vi "lorentzian transformations.vi"(6 "factor":dbl=1.0, 7 "4 corner circle transformation":T3=enum."fix phase", 8 "lorentzian in":T2 {"z∞ (V)" format="%#_4p"; "Q" format="%#_4p"; "φ (rad)" format="%#_3p"; "Γ (Hz)" format="%#_5p"; "ω (Hz)" format="%#_9p"; "A (VHz)" format="%#_3p"}, 9 "phase in (rad)":dbl, 10 "freq in":dbl, 11 "voltage in":cdb) -> (0 "lorentzian out":T2={"A (VHz)"=-1.0311345636926572, "ω (Hz)"=-1.0311345636926572, "Γ (Hz)"=-1.0311345636926572, "φ (rad)"=-1.0311345636926572, "Q"=-1.0311345636926572, "Norm  Ampl"=-1.0311345636926572, "z∞ (V)"=-1.0311345636926572+0.0i, "4corners"={"z (-pi/2)"=-1.0311345636926572+0.5736824521422934i, "z(inf)"=-0.5200164984937075+1.0975277942502903i, "z (pi/2)"=-1.0311345636926572+0.5736824521422934i, "z center"=-0.5136528600391839+0.580046090596817i, "z(0)"=-0.5200164984937075+1.0975277942502903i, "radius"=-1.0311345636926572}} {"z∞ (V)" format="%#_4p"; "Q" format="%#_4p"; "φ (rad)" format="%#_3p"; "Γ (Hz)" format="%#_5p"; "ω (Hz)" format="%#_9p"; "A (VHz)" format="%#_3p"}, 1 "4corners our":T1={"z (-pi/2)"=-1.0311345636926572+0.5736824521422934i, "z(inf)"=-0.5200164984937075+1.0975277942502903i, "z (pi/2)"=-1.0311345636926572+0.5736824521422934i, "z center"=-0.5136528600391839+0.580046090596817i, "z(0)"=-0.5200164984937075+1.0975277942502903i, "radius"=-1.0311345636926572}, 2 "gamma OUT":dbl, 3 "voltage out":cdb)   [LabVIEW 2020]
uses:
  four-corner circle transformation.ctl
  lorentzian.ctl
  circle corners.ctl
  Q - not nan -- real.vi
panel:
  out "freq OUT":dbl
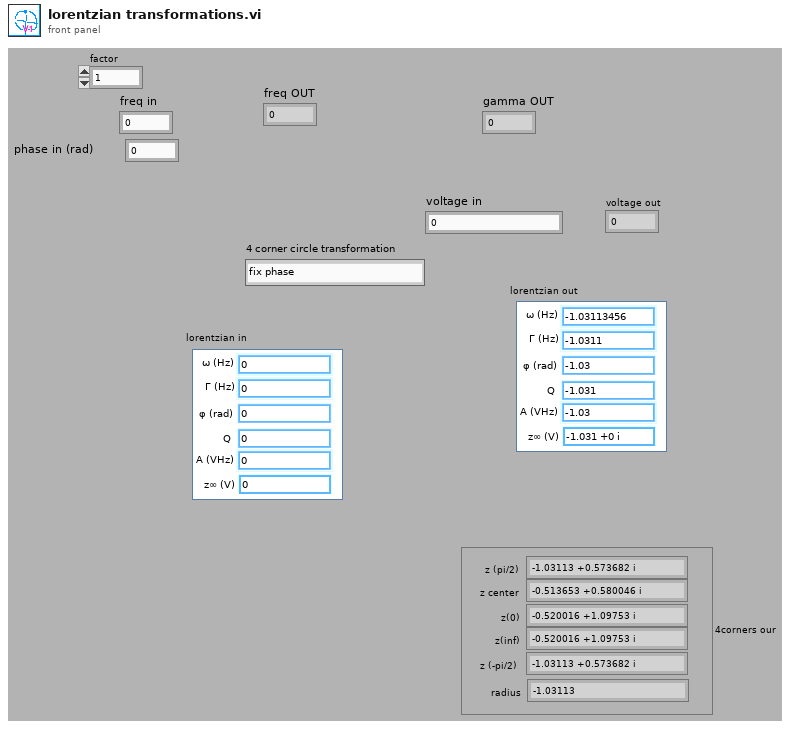
[diagram p1: front panel]
types:
  T1 = typedef "circle corners.ctl" = cluster{"z (-pi/2)":cdb, "z(inf)":cdb, "z (pi/2)":cdb, "z center":cdb, "z(0)":cdb, "radius":dbl}
  T2 = typedef "lorentzian.ctl" = cluster{"A (VHz)":dbl, "ω (Hz)":dbl, "Γ (Hz)":dbl, "φ (rad)":dbl, "Q":dbl, "Norm  Ampl":dbl, "z∞ (V)":cdb, "4corners":T1}
  T3 = typedef "four-corner circle transformation.ctl" = enum16{"z(c) z(inf)", "z(c) z(zero)", "fix phase", "calculate lorentzian", "z(0) z(+-pi/2)", "shift to zcenter", "to  canonical", "get canonical phase", "get4corners", "update lorentzian -- from z0", "fake gamma normal", "fake gamma heat", "calculate complex slope", "get f0 given f and phi"}
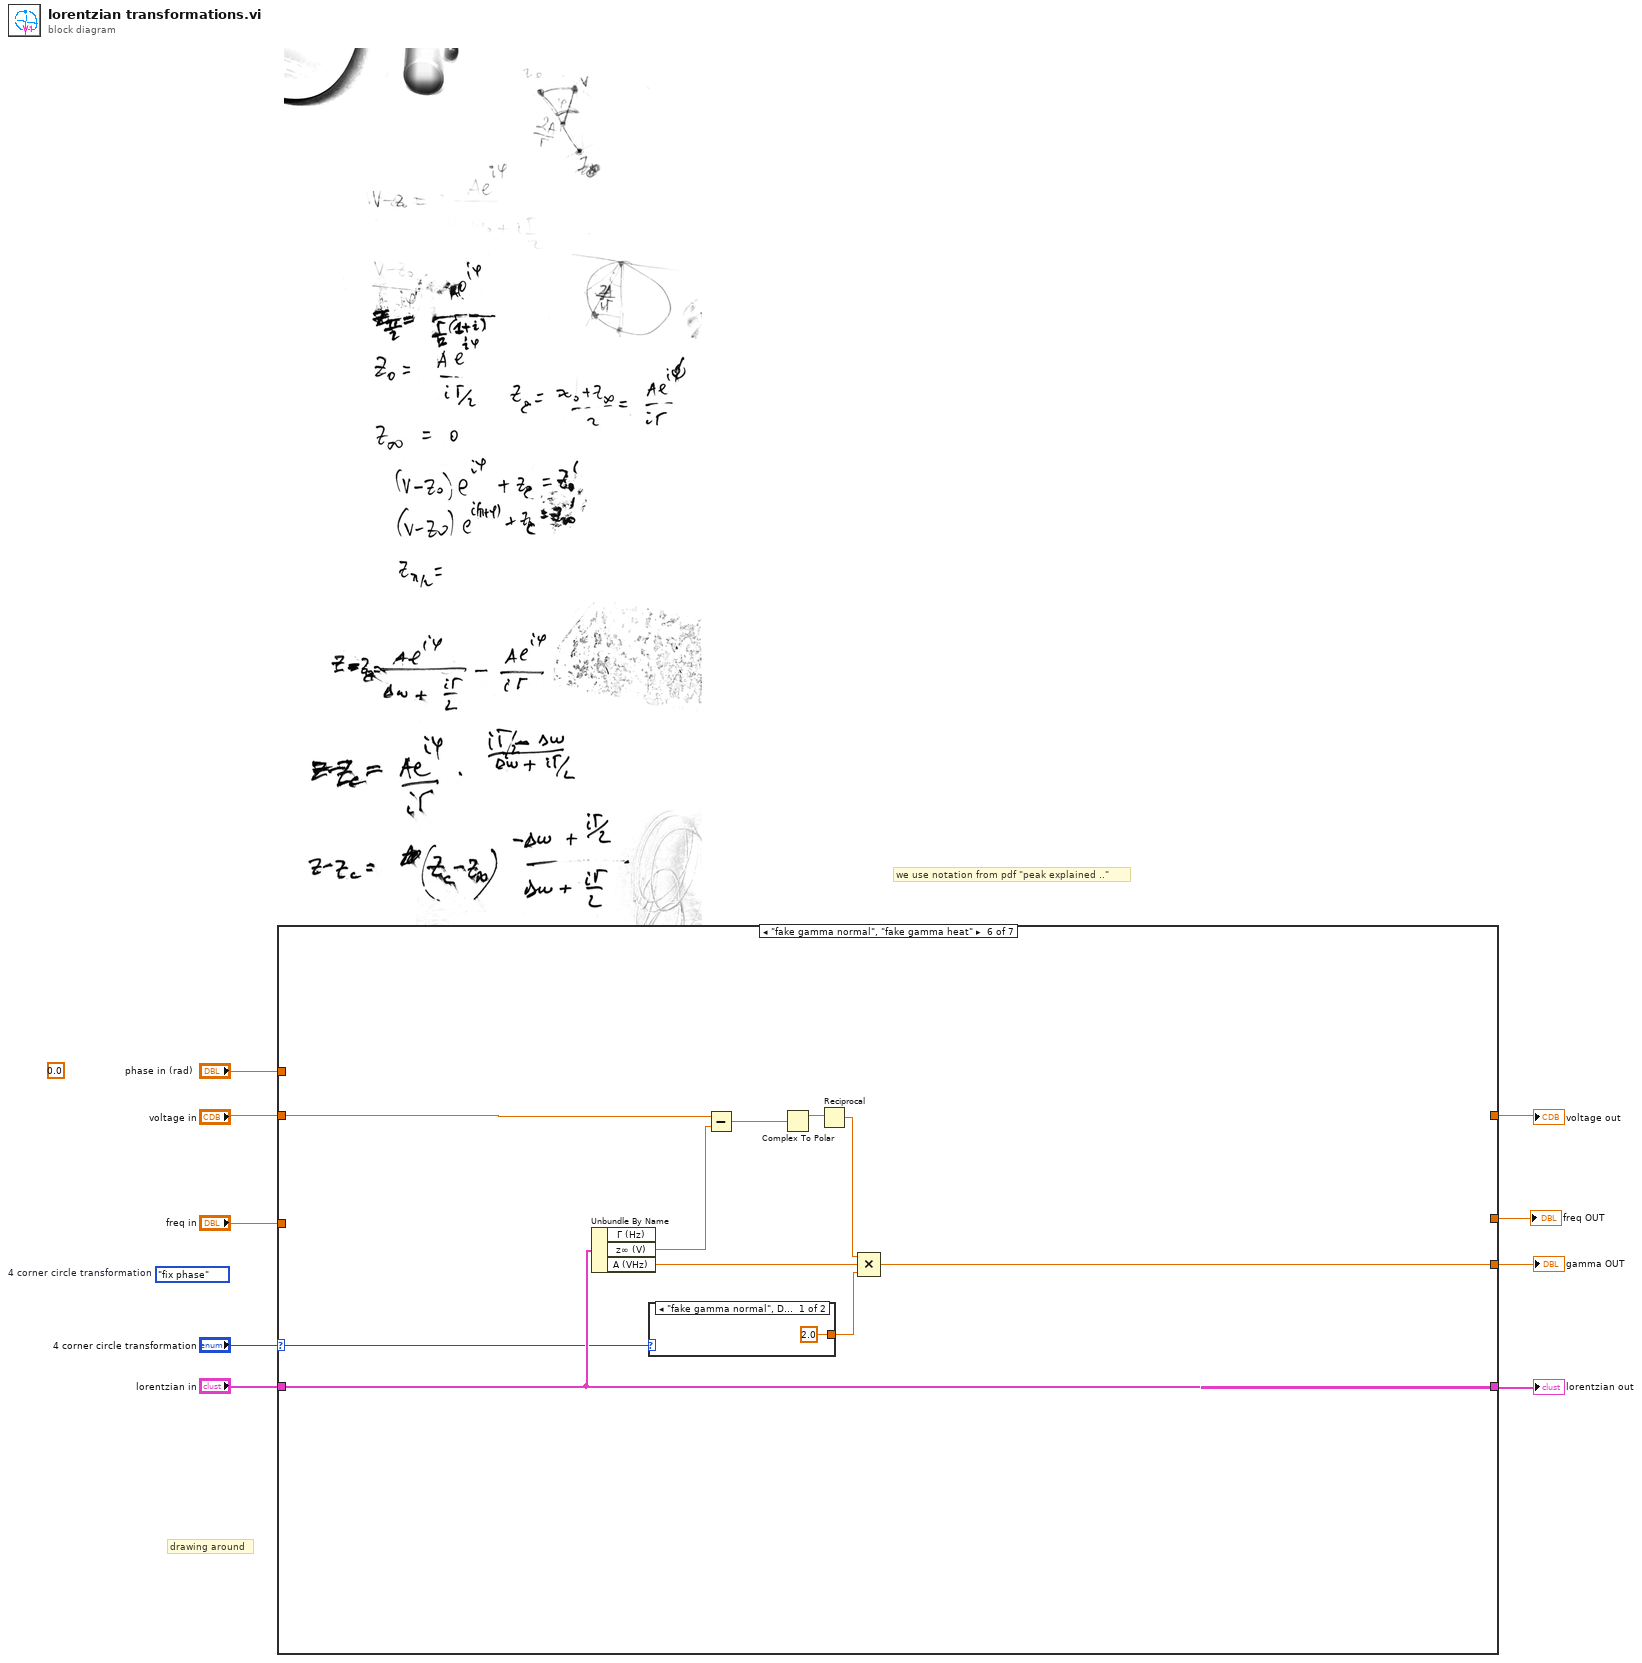
[diagram p0: block diagram]
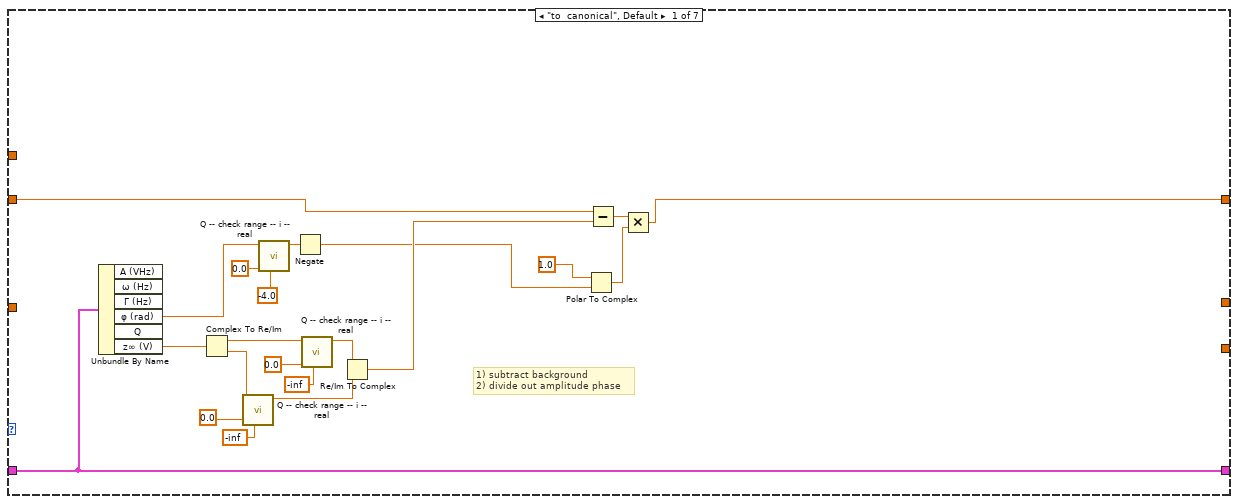
[diagram p2: hidden frame]
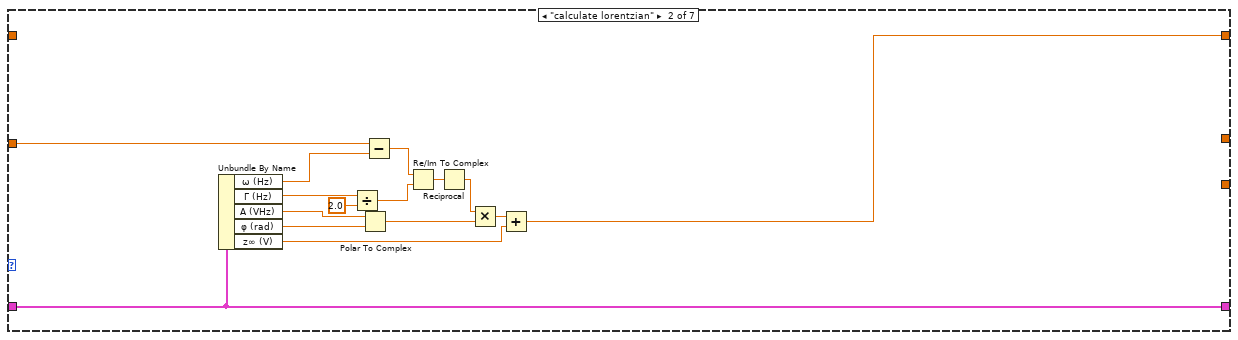
[diagram p3: hidden frame]
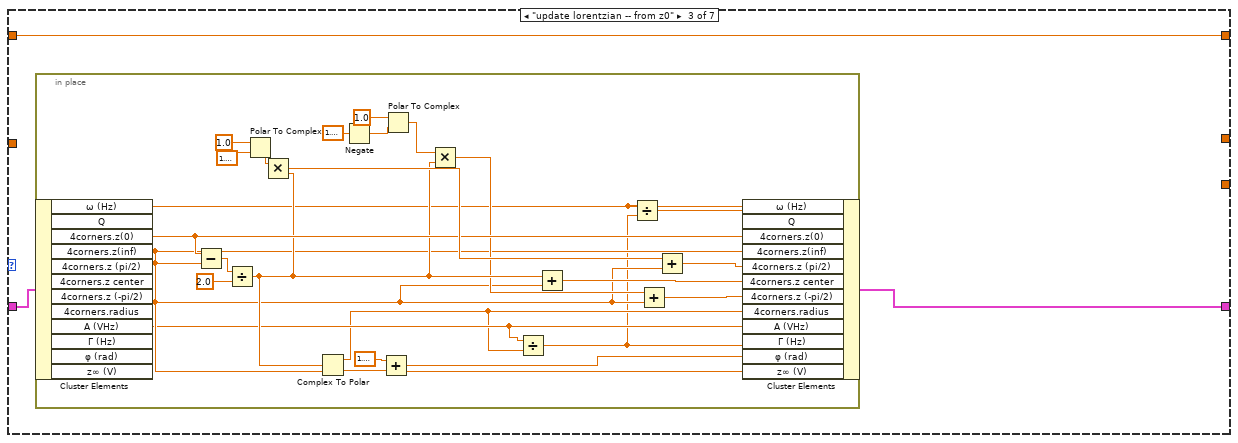
[diagram p4: hidden frame]
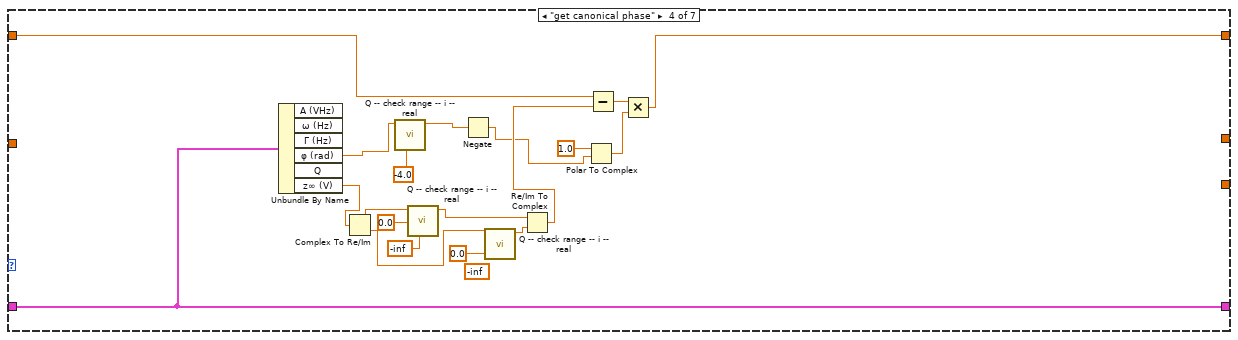
[diagram p5: hidden frame]
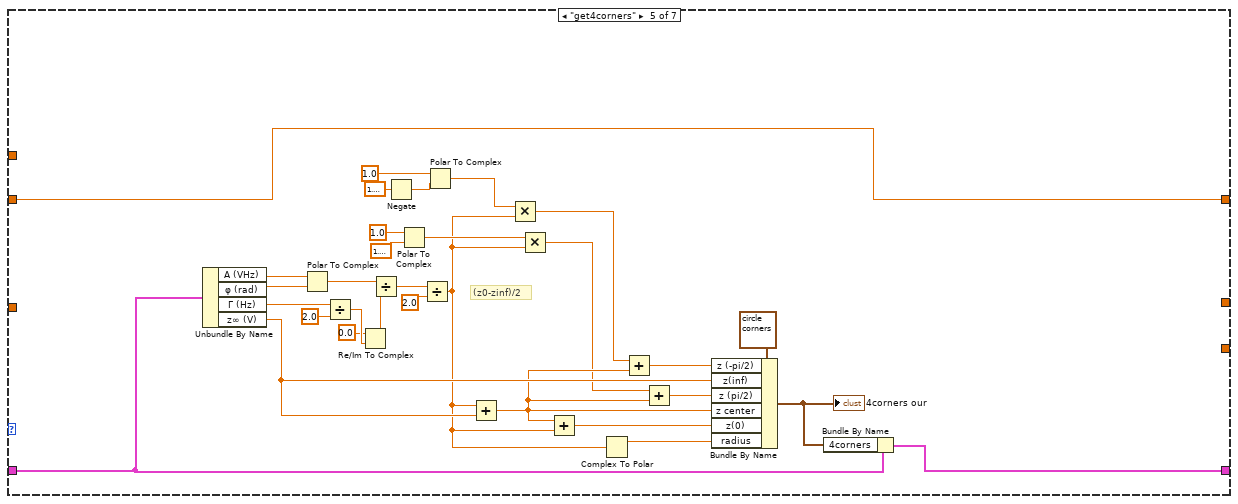
[diagram p6: hidden frame]
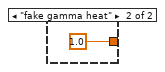
[diagram p7: hidden frame]
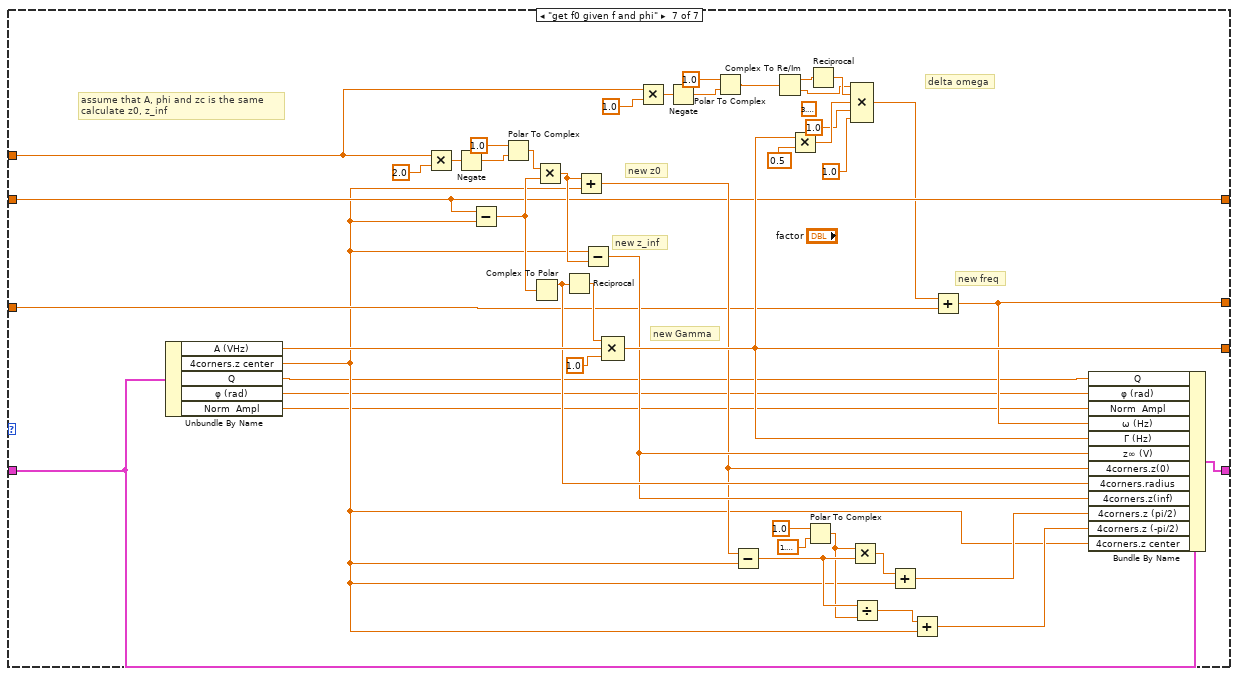
[diagram p8: hidden frame]
diagram:
  (unwired) 0.0 ("zi phase temporary")
  (unwired) four-corner_circle_transformation."fix phase"  # 4 corner circle transformation
  # "we use notation from pdf \"peak explained ..\""
  # "drawing around"
  n1 = case shown="\"fake gamma normal\", \"fake gamma heat\"" "4 corner circle transformation" {
    selector: "4 corner circle transformation" -> [_ _ _ _ _ w124 _]
    tunnel: "voltage in" -> [w13 _ w46 w75 w102 w127 w153]
    tunnel: [w14 w45 w47 w76 w95 w126 w171] -> w7
    tunnel: "lorentzian in" -> [w14 w45 w48 w76 w97 w126 w172]
    tunnel: [w12 w39 w46 w74 w102 _ w153] -> w5
    tunnel: "freq in" -> [_ w44 _ _ _ _ w152]
    tunnel: [_ _ _ _ _ w125 w168] -> w3
    tunnel: "phase in (rad)" -> [_ _ _ _ _ _ w146]
    tunnel: [_ _ _ _ _ _ w154] -> w1
    frame "to  canonical", Default {
      # "1) subtract background\n2) divide out amplitude phase"
      n2 = Unbundle By Name(w14) -> ("φ (rad)"=w27:dbl, "z∞ (V)"=w25:cdb)  [unwired: 4 out]
      n3 = Complex To Re/Im(x + iy=w25) -> (x=w24:dbl, y=w22:dbl)
      n4 = call "Q -- check range -- i -- real.vi"("lower"=-inf, "default"=0.0, "number"=w22) -> ("number in range"=w19:dbl)  [unwired: 6 in, 2 out]
      n5 = call "Q -- check range -- i -- real.vi"("lower"=-4.0, "default"=0.0, "number"=w27) -> ("number in range"=w16:dbl)  [unwired: 6 in, 2 out]
      n6 = Negate(x=w16) -> (-x=w15:dbl)
      n7 = call "Q -- check range -- i -- real.vi"("lower"=-inf, "default"=0.0, "number"=w24) -> ("number in range"=w18:dbl)  [unwired: 6 in, 2 out]
      n8 = Re/Im To Complex(1:w19, 2:w18) -> (0:w17:cdb)
      n9 = Polar To Complex(1:w15, 2:1.0 ("r")) -> (0:w28:cdb)
      n10 = Subtract(x=w13, y=w17) -> (x-y=w29:cdb)
      n11 = Multiply(x=w29, y=w28) -> (x*y=w12:cdb)
    }
    frame "calculate lorentzian" {
      n12 = Unbundle By Name(w45) -> ("ω (Hz)"=w32:dbl, "Γ (Hz)"=w31:dbl, "A (VHz)"=w33:dbl, "φ (rad)"=w43:dbl, "z∞ (V)"=w40:cdb)
      n13 = Divide(x=w31, y=2.0 ("x")) -> (x/y=w35:dbl)
      n14 = Polar To Complex(1:w43, 2:w33) -> (0:w42:cdb)
      n15 = Subtract(x=w44, y=w32) -> (x-y=w37:dbl)
      n16 = Re/Im To Complex(1:w35, 2:w37) -> (0:w34:cdb)
      n17 = Reciprocal(x=w34) -> (1/x=w38:cdb)
      n18 = Multiply(x=w38, y=w42) -> (x*y=w41:cdb)
      n19 = Add(x=w41, y=w40) -> (x+y=w39:cdb)
    }
    frame "update lorentzian -- from z0" {
      n20 = in-place {
        n21 = in-place-cluster #1(w48) -> ("ω (Hz)"=w51:dbl, "4corners.z(0)"=w58:cdb, "4corners.z(inf)"=w54:cdb, "A (VHz)"=w53:dbl)  [unwired: 8 out]
        n22 = Subtract(x=w58, y=w54) -> (x-y=w69:cdb)
        n23 = Divide(x=w69, y=2.0) -> (x/y=w57:cdb)
        n24 = Polar To Complex(1:1.5707963267948966, 2:1.0 ("r")) -> (0:w62:cdb)
        n25 = Multiply(x=w62, y=w57) -> (x*y=w60:cdb)
        n26 = Complex To Polar(r * e^(i*theta)=w57) -> (r=w52:dbl, theta=w72:dbl)
        n27 = Negate(x=1.5707963267948966) -> (-x=w63:dbl)
        n28 = Add(x=1.5707963267948966, y=w72) -> (x+y=w71:dbl)
        n29 = Polar To Complex(1:w63, 2:1.0 ("r")) -> (0:w61:cdb)
        n30 = Multiply(x=w61, y=w57) -> (x*y=w56:cdb)
        n31 = Divide(x=w53, y=w52) -> (x/y=w50:dbl)
        n32 = Add(x=w57, y=w54) -> (x+y=w68:cdb)
        n33 = Divide(x=w51, y=w50) -> (x/y=w49:dbl)
        n34 = Add(x=w56, y=w54) -> (x+y=w55:cdb)
        n35 = Add(x=w60, y=w54) -> (x+y=w59:cdb)
        n36 = in-place-cluster #1("ω (Hz)"=w51, "Q"=w49, "4corners.z(0)"=w58, "4corners.z(inf)"=w54, "4corners.z (pi/2)"=w59, "4corners.z center"=w68, "4corners.z (-pi/2)"=w55, "4corners.radius"=w52, "A (VHz)"=w53, "Γ (Hz)"=w50, "φ (rad)"=w71, "z∞ (V)"=w54) -> (w47:T2)
      }
    }
    frame "get canonical phase" {
      (unwired) -inf ("lower")
      n37 = Unbundle By Name(w76) -> ("φ (rad)"=w89:dbl, "z∞ (V)"=w87:cdb)  [unwired: 4 out]
      n38 = Complex To Re/Im(x + iy=w87) -> (x=w86:dbl, y=w84:dbl)
      n39 = call "Q -- check range -- i -- real.vi"("lower"=-4.0, "number"=w89) -> ("number in range"=w78:dbl)  [unwired: 7 in, 2 out]
      n40 = call "Q -- check range -- i -- real.vi"("lower"=-inf, "default"=0.0, "number"=w86) -> ("number in range"=w80:dbl)  [unwired: 6 in, 2 out]
      n41 = Negate(x=w78) -> (-x=w77:dbl)
      n42 = call "Q -- check range -- i -- real.vi"("default"=0.0, "number"=w84) -> ("number in range"=w81:dbl)  [unwired: 7 in, 2 out]
      n43 = Re/Im To Complex(1:w81, 2:w80) -> (0:w79:cdb)
      n44 = Polar To Complex(1:w77, 2:1.0 ("r")) -> (0:w90:cdb)
      n45 = Subtract(x=w75, y=w79) -> (x-y=w91:cdb)
      n46 = Multiply(x=w91, y=w90) -> (x*y=w74:cdb)
    }
    frame "get4corners" {
      # "(z0-zinf)/2"
      n47 = Unbundle By Name(w97) -> ("A (VHz)"=w122:dbl, "φ (rad)"=w121:dbl, "Γ (Hz)"=w119:dbl, "z∞ (V)"=w108:cdb)
      n48 = Polar To Complex(1:w121, 2:w122) -> (0:w118:cdb)
      n49 = Divide(x=w119, y=2.0) -> (x/y=w105:dbl)
      n50 = Re/Im To Complex(1:w105, 2:0.0 ("x")) -> (0:w103:cdb)
      n51 = Divide(x=w118, y=w103) -> (x/y=w109:cdb)
      n52 = Negate(x=1.5707963267948966) -> (-x=w111:dbl)
      n53 = Polar To Complex(1:1.5707963267948966, 2:1.0 ("r")) -> (0:w107:cdb)
      n54 = Divide(x=w109, y=2.0) -> (x/y=w98:cdb)
      n55 = Polar To Complex(1:w111, 2:1.0 ("r")) -> (0:w106:cdb)
      n56 = Add(x=w98, y=w108) -> (x+y=w99:cdb)
      n57 = Multiply(x=w106, y=w98) -> (x*y=w94:cdb)
      n58 = Multiply(x=w107, y=w98) -> (x*y=w93:cdb)
      n59 = Add(x=w99, y=w98) -> (x+y=w117:cdb)
      n60 = Complex To Polar(r * e^(i*theta)=w98) -> (r=w116:dbl)  [unwired: 1 out]
      n61 = Add(x=w94, y=w99) -> (x+y=w101:cdb)
      n62 = Add(x=w93, y=w99) -> (x+y=w100:cdb)
      n63 = Bundle By Name(cluster=T1 {"z (-pi/2)"=-1.0311345636926572+0.5736824521422934i, "z(inf)"=-0.5200164984937075+1.0975277942502903i, "z (pi/2)"=-1.0311345636926572+0.5736824521422934i, "z center"=-0.5136528600391839+0.580046090596817i, "z(0)"=-0.5200164984937075+1.0975277942502903i, "radius"=-1.0311345636926572} ("circle corners"), "z (-pi/2)"=w101, "z(inf)"=w108, "z (pi/2)"=w100, "z center"=w99, "z(0)"=w117, "radius"=w116) -> (w96:T1)
      "4corners our" <- w96
      n64 = Bundle By Name(cluster=w97, "4corners"=w96) -> (w95:T2)
    }
    frame "fake gamma normal", "fake gamma heat" {
      n65 = Unbundle By Name(w126) -> ("z∞ (V)"=w129:cdb, "A (VHz)"=w128:dbl)  [unwired: 1 out]
      n66 = case shown="\"fake gamma normal\", Default" w124 {
        tunnel: [2.0 ("value") 1.0 ("value")] -> w133
        frame "fake gamma normal", Default {
        }
        frame "fake gamma heat" {
        }
      }
      n67 = Subtract(x=w127, y=w129) -> (x-y=w132:cdb)
      n68 = Complex To Polar(r * e^(i*theta)=w132) -> (r=w131:dbl)  [unwired: 1 out]
      n69 = Reciprocal(x=w131) -> (1/x=w130:dbl)
      n70 = Compound Arithmetic op=MULTIPLY(w130, w128, w133) -> (w125:dbl)
    }
    frame "get f0 given f and phi" {
      (unwired) 3.141592653589793
      # "new freq"
      # "delta omega"
      # "new Gamma"
      # "new z_inf"
      # "new z0"
      # "assume that A, phi and zc is the same \ncalculate z0, z_inf"
      n71 = Unbundle By Name(w172) -> ("A (VHz)"=w180:dbl, "4corners.z center"=w141:cdb, "Q"=w138:dbl, "φ (rad)"=w139:dbl, "Norm  Ampl"=w140:dbl)
      n72 = Multiply(x=w146, y=2.0) -> (x*y=w173:dbl)
      n73 = Negate(x=w173) -> (-x=w151:dbl)
      n74 = Subtract(x=w153, y=w141) -> (x-y=w177:cdb)
      n75 = Polar To Complex(1:w151, 2:1.0 ("r")) -> (0:w166:cdb)
      n76 = Complex To Polar(r * e^(i*theta)=w177) -> (r=w169:dbl)  [unwired: 1 out]
      n77 = Multiply(x=w166, y=w177) -> (x*y=w178:cdb)
      n78 = Reciprocal(x=w169) -> (1/x=w175:dbl)
      n79 = Add(x=w178, y=w141) -> (x+y=w163:cdb)
      n80 = Subtract(x=w141, y=w178) -> (x-y=w167:cdb)
      n81 = Compound Arithmetic op=MULTIPLY(w175, w180, 1.0 ("value")) -> (w168:dbl)
      n82 = Multiply(x=w146, y=1.0) -> (x*y=w148:dbl)
      n83 = Negate(x=w148) -> (-x=w147:dbl)
      n84 = Polar To Complex(1:w147, 2:1.0 ("r")) -> (0:w145:cdb)
      n85 = Subtract(x=w163, y=w141) -> (x-y=w158:cdb)
      n86 = Complex To Re/Im(x + iy=w145) -> (x=w144:dbl, y=w143:dbl)
      n87 = Multiply(x=w168, y=0.5) -> (x*y=w164:dbl)
      n88 = Polar To Complex(1:1.5707963267948966, 2:1.0 ("r")) -> (0:w157:cdb)
      n89 = Reciprocal(x=w144) -> (1/x=w165:dbl)
      n90 = Multiply(x=w157, y=w158) -> (x*y=w160:cdb)
      n91 = Compound Arithmetic op=MULTIPLY(w143, w165, w164, 1.0 ("value"), 1.0 ("value")) -> (w142:dbl)
      n92 = Divide(x=w158, y=w157) -> (x/y=w156:cdb)
      n93 = Add(x=w160, y=w141) -> (x+y=w159:cdb)
      n94 = Add(x=w156, y=w141) -> (x+y=w155:cdb)
      n95 = Add(x=w142, y=w152) -> (x+y=w154:dbl)
      n96 = Bundle By Name(cluster=w172, "Q"=w138, "φ (rad)"=w139, "Norm  Ampl"=w140, "ω (Hz)"=w154, "Γ (Hz)"=w168, "z∞ (V)"=w167, "4corners.z(0)"=w163, "4corners.radius"=w169, "4corners.z(inf)"=w167, "4corners.z (pi/2)"=w159, "4corners.z (-pi/2)"=w155, "4corners.z center"=w141) -> (w171:T2)
    }
  }
  "lorentzian out" <- w7
  "voltage out" <- w5
  "freq OUT" <- w1
  "gamma OUT" <- w3
